vi "Scale Graphs.vi"(4 "IGain":dbl=4.0, 5 "I Scale":dbl(slide) min=-6.0 max=0.0 step=1.0 scale=0.0..-6.0, 6 "VGain":dbl=4.0, 7 "V Scale":dbl(slide) min=-6.0 max=0.0 step=1.0 scale=0.0..-6.0, 9 "IR (ohms)":dbl=4.0, 10 "Channel 0 (Current)":dbl=4.0, 11 "Wfm Data":waveform(dbl)[](graph)) -> (0 "DAQ Input":waveform(dbl)[](graph), 2 "Scaled Wfm (I,V)":waveform(dbl)[](graph), 3 "Wfm (I,V)":waveform(dbl)[](graph))   [LabVIEW 2018]
panel:
  # "Input"
  # "Output"
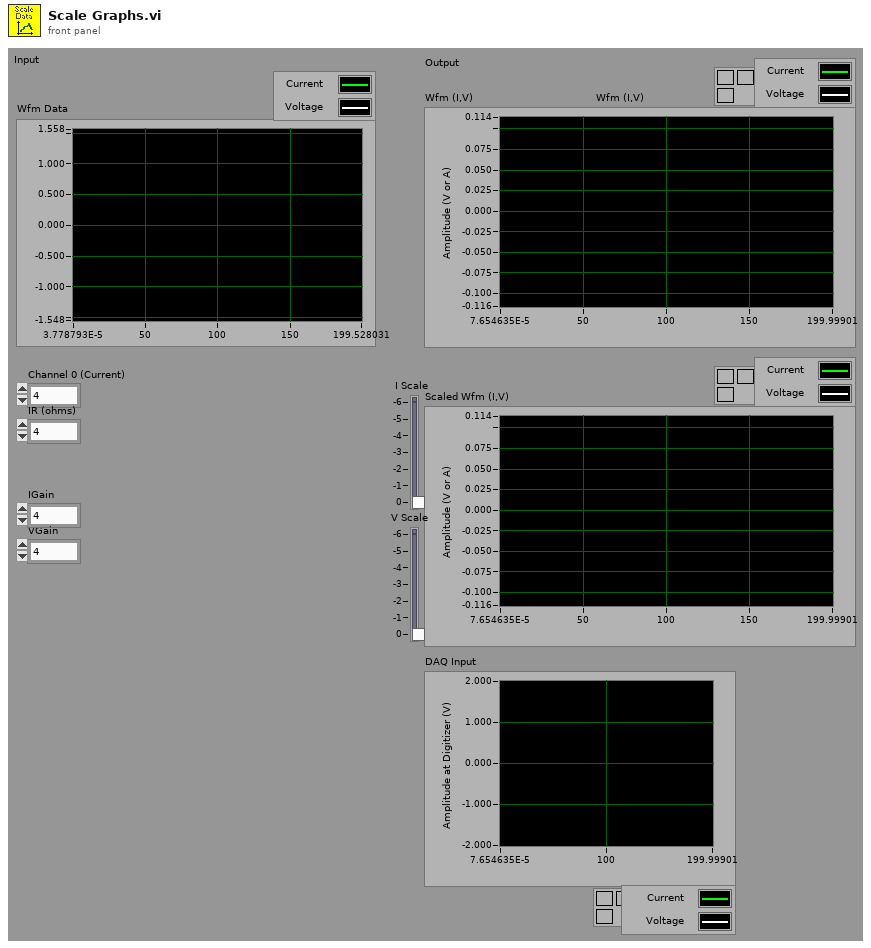
[diagram p1: front panel]
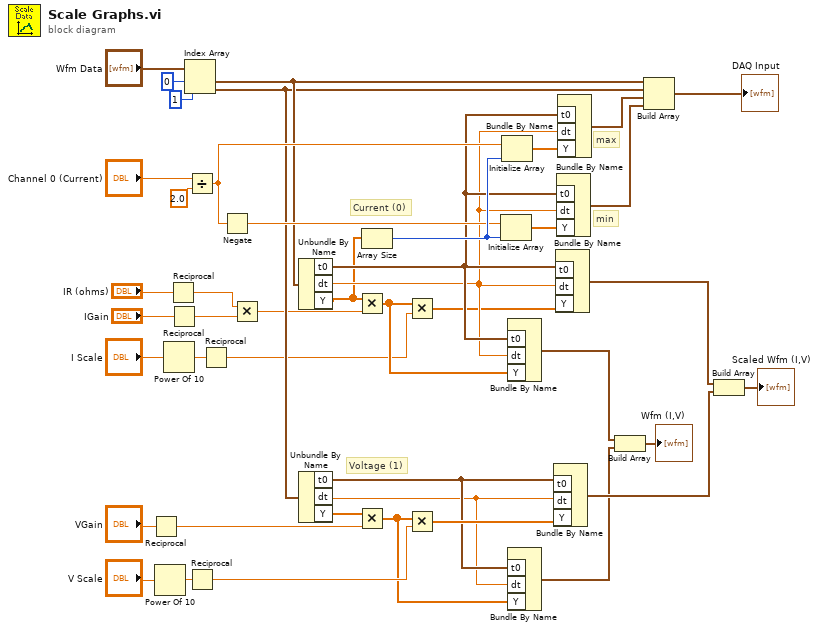
[diagram p0: block diagram]
diagram:
  # "Voltage (1)"
  # "Current (0)"
  # "min"
  # "max"
  n1 = Reciprocal(x="VGain") -> (1/x=w6:dbl)
  n2 = Power Of 10(x="V Scale") -> (10^x=w38:dbl)
  n3 = Power Of 10(x="I Scale") -> (10^x=w37:dbl)
  n4 = Reciprocal(x="IR (ohms)") -> (1/x=w13:dbl)
  n5 = Reciprocal(x="IGain") -> (1/x=w12:dbl)
  n6 = Index Array(array="Wfm Data", index #1=0 ("index"), index #2=1 ("index")) -> (element #1=w27:waveform(dbl), element #2=w21:waveform(dbl))
  n7 = Divide(x="Channel 0 (Current)", y=2.0 ("x")) -> (x/y=w32:dbl)
  n8 = Reciprocal(x=w38) -> (1/x=w5:dbl)
  n9 = Reciprocal(x=w37) -> (1/x=w10:dbl)
  n10 = Negate(x=w32) -> (-x=w35:dbl)
  n11 = Multiply(x=w13, y=w12) -> (x*y=w14:dbl)
  n12 = Unbundle By Name(w27) -> ("t0"=w17:timestamp, "dt"=w16:dbl, "Y"=w15:dbl[])
  n13 = Unbundle By Name(w21) -> ("t0"=w3:timestamp, "dt"=w2:dbl, "Y"=w20:dbl[])
  n14 = Multiply(x=w15, y=w14) -> (x*y=w11:dbl[])
  n15 = Multiply(x=w20, y=w6) -> (x*y=w1:dbl[])
  n16 = Array Size(array=w15) -> (size(s)=w39:i32)
  n17 = Multiply(x=w11, y=w10) -> (x*y=w9:dbl[])
  n18 = Multiply(x=w1, y=w5) -> (x*y=w4:dbl[])
  n19 = Initialize Array(w35, w39) -> (w23:dbl[])
  n20 = Initialize Array(w32, w39) -> (w25:dbl[])
  n21 = Bundle By Name("t0"=w17, "dt"=w16, "Y"=w11) -> (w8:waveform(dbl))  [unwired: 1 in]
  n22 = Bundle By Name("t0"=w3, "dt"=w2, "Y"=w1) -> (w7:waveform(dbl))  [unwired: 1 in]
  n23 = Bundle By Name("t0"=w3, "dt"=w2, "Y"=w4) -> (w19:waveform(dbl))  [unwired: 1 in]
  n24 = Bundle By Name("t0"=w17, "dt"=w16, "Y"=w9) -> (w22:waveform(dbl))  [unwired: 1 in]
  n25 = Bundle By Name("t0"=w17, "dt"=w16, "Y"=w23) -> (w24:waveform(dbl))  [unwired: 1 in]
  n26 = Bundle By Name("t0"=w17, "dt"=w16, "Y"=w25) -> (w26:waveform(dbl))  [unwired: 1 in]
  n27 = Build Array(w8, w7) -> (→"Wfm (I,V)":waveform(dbl)[])
  n28 = Build Array(w27, w21, w26, w24) -> (→"DAQ Input":waveform(dbl)[])
  n29 = Build Array(w22, w19) -> (→"Scaled Wfm (I,V)":waveform(dbl)[])
